vi "SIM update timestep base.vi"(5 "Timestep Index":dbl, 6 "current timestep base":dbl, 7 "step size":dbl) -> (1 "Timestep Index out":dbl, 2 "current timestep base out":dbl)   [LabVIEW 2018]
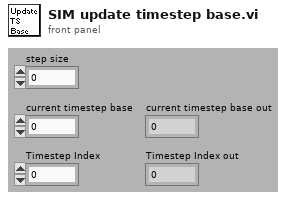
[diagram p1: front panel]
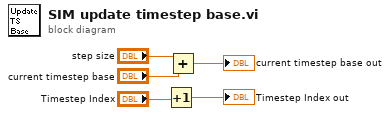
[diagram p0: block diagram]
diagram:
  n1 = Increment(x="Timestep Index") -> (x+1=→"Timestep Index out":dbl)
  n2 = Add(x="step size", y="current timestep base") -> (x+y=→"current timestep base out":dbl)
